vi "Get Channel List.vi"(8 "error in (no error)":errorcluster, 10 "Slave resource names":string[](array[string]), 11 "Master resouce name":string) -> (0 "error out":errorcluster, 3 "Channel List":T1[](array[typedef]))   [LabVIEW 2021]
uses:
  ctl/NIDCPower_channel_ganging - ctl - channel def.ctl
  ctl/NIDCPower_channel_ganging - ctl - channel mode.ctl
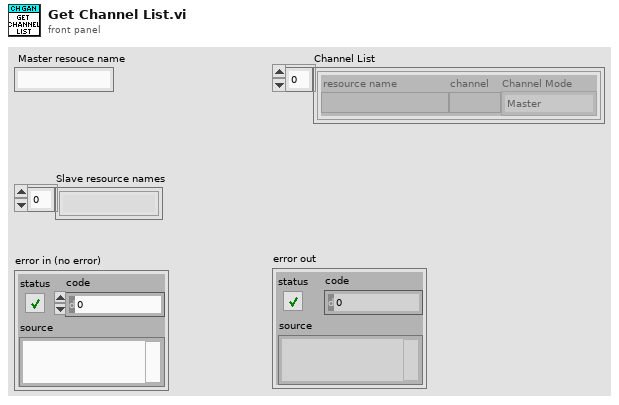
[diagram p1: front panel]
types:
  T1 = typedef "NIDCPower_channel_ganging - ctl - channel def.ctl" = cluster{"resource name":refnum<k15>, "channels":string, "Channel Mode":T2}
  T2 = typedef "NIDCPower_channel_ganging - ctl - channel mode.ctl" = enum32{"Master", "Slave", "Slave - Inverted"}
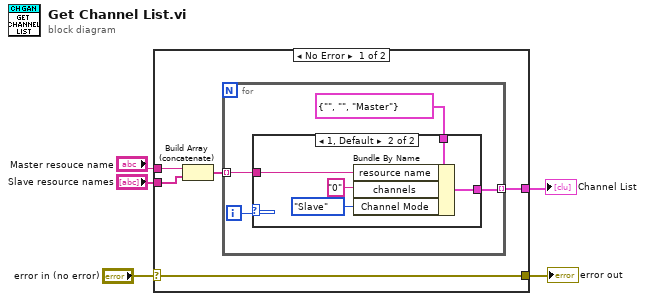
[diagram p0: block diagram]
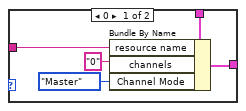
[diagram p2: hidden frame]
diagram:
  n1 = case shown="No Error" "error in (no error)" {
    selector: "error in (no error)" -> [w6 w25]
    tunnel: "Slave resource names" -> [w9 _]
    tunnel: "Master resouce name" -> [w8 _]
    tunnel: [w7 _] -> w3
    tunnel: [w6 w25] -> w1
    frame No Error {
      n2 = Build Array (concatenate)(w8, w9) -> (w10:string[])
      n3 = for {
        tunnel: [w14] -> w7 mode=indexing
        tunnel: w10 -> [w12] mode=indexing
        i -> [w13]
        n4 = case shown="1, Default" w13 {
          tunnel: [w19 w24] -> w14
          tunnel: w12 -> [w16 w21]
          tunnel: T1 {"resource name"="", "channels"="", "Channel Mode"=enum."Master"} ("Channel Def") -> [w15 w20]
          frame 0 {
            n5 = Bundle By Name(cluster=w15, "resource name"=w16, "channels"="0", "Channel Mode"=NIDCPower_channel_ganging_-_ctl_-_channel_mode."Master") -> (w19:T1)
          }
          frame 1, Default {
            n6 = Bundle By Name(cluster=w20, "resource name"=w21, "channels"="0", "Channel Mode"=NIDCPower_channel_ganging_-_ctl_-_channel_mode."Slave") -> (w24:T1)
          }
        }
      }
    }
    frame Error {
    }
  }
  "Channel List" <- w3
  "error out" <- w1
